vi "Execute Test.vi"(8 "error in (no error)":errorcluster, 9 "Processing":refnum<queue>, 10 "UI in":refnum<queue>, 11 "Settings in":T1 {"Processing Settings"."Test Parameters"."Allowed Tolerance (%) FS" format="%#_4g"; "Acq Settings"."Config Settings"."Simulated Sensor Injection" scale=0.0..100.0}) -> (0 "error out":errorcluster, 2 "UI out":refnum<queue>, 3 "Settings out":T1 {"Processing Settings"."Test Parameters"."Allowed Tolerance (%) FS" format="%#_4g"; "Acq Settings"."Config Settings"."Simulated Sensor Injection" scale=0.0..100.0})   [LabVIEW 2026]
uses:
  controls/UI/Settings Cluster.ctl
  controls/UI/Acq Settings.ctl
  Acquisition/Instrument Specifications Configuration.ctl
  Acquisition/Instrument Specifications Cluster Configuration.ctl
  controls/UI/Measurement Role.ctl
  controls/UI/Config Settings.ctl
  Processing/Processing Settings.ctl
  controls/Messaging Payloads/Sensor CoreData.ctl
  controls/Messaging Payloads/Sensor CoreData Cluster.ctl
  controls/UI/Units Enum.ctl
  controls/UI/Signal Enum.ctl
  Processing/Test Parameters.ctl
  Processing/Test Parameters Cluster.ctl
  controls/UI/Test Sequence Context.ctl
  controls/UI/Direction.ctl
  controls/UI/Session Identfiers.ctl
  controls/UI/Test Sequence Settings.ctl
  controls/UI/Test Sequence State.ctl
  controls/UI/Test Sequence Enum.ctl
  controls/Controller/Stimulus Settings.ctl
  controls/Controller/Stimulus Outputs.ctl
  controls/Controller/Stimulus Output.ctl
  controls/Controller/Controller Core Data.ctl
  controls/Controller/Stimulus Output Configuration.ctl
  controls/Controller/Stimulus Role.ctl
  Architecture/Message Queue/Message Cluster.ctl
  Architecture/Message Queue/Enqueue Message (Single).vi
  Architecture/Message Queue/Message Queue.lvlib
  Settings/Settings.lvlib
  Acquisition/Acquisition.lvlib
  Processing/Processing_Engine.lvlib
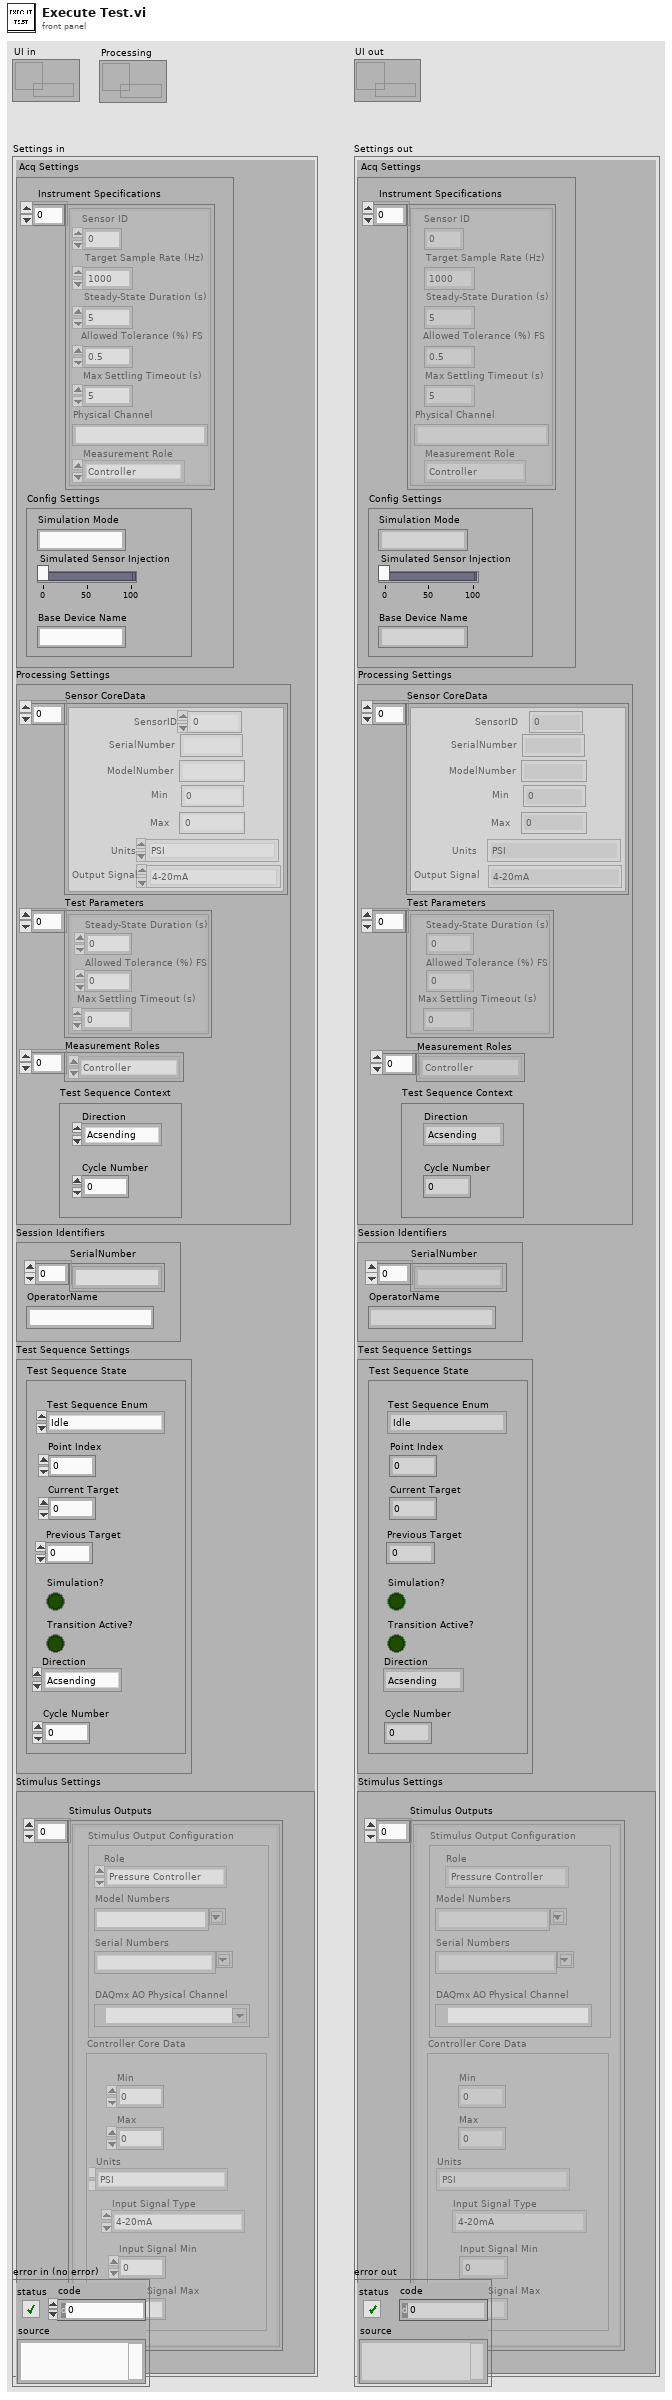
[diagram p1: front panel]
types:
  T1 = typedef "Settings Cluster.ctl" = cluster{"Acq Settings":T2, "Processing Settings":T7, "Session Identifiers":T16, "Test Sequence Settings":T17, "Stimulus Settings":T20}
  T2 = typedef "Acq Settings.ctl" = cluster{"Instrument Specifications":T3, "Config Settings":T6}
  T3 = typedef "Acquisition.lvlib/Instrument Specifications Configuration.ctl" = T4[]
  T4 = typedef "Acquisition.lvlib/Instrument Specifications Cluster Configuration.ctl" = cluster{"Sensor ID":i32, "Target Sample Rate (Hz)":dbl, "Steady-State Duration (s)":i32, "Allowed Tolerance (%) FS":dbl, "Max Settling Timeout (s)":i32, "Physical Channel":string, "Measurement Role":T5}
  T5 = typedef "Settings.lvlib/Measurement Role.ctl" = enum16{"Controller", "Reference", "UUT", "Disable", "All"}
  T6 = typedef "Config Settings.ctl" = cluster{"Simulated Sensor Injection":dbl, "Base Device Name":string, "Simulation Mode":string}
  T7 = typedef "Processing_Engine.lvlib/Processing Settings.ctl" = cluster{"Sensor CoreData":T8, "Test Parameters":T12, "Measurement Roles":T5[], "Test Sequence Context":T14}
  T8 = typedef "Sensor CoreData.ctl" = T9[]
  T9 = typedef "Settings.lvlib/Sensor CoreData Cluster.ctl" = cluster{"SerialNumber":string, "ModelNumber":string, "Min":dbl, "Max":dbl, "Units":T10, "Output Signal":T11, "SensorID":i32}
  T10 = typedef "Units Enum.ctl" = enum16{"PSI", "Deg C", "kPa", "GPM"}
  T11 = typedef "Signal Enum.ctl" = enum16{"4-20mA", "0-10V", "Thermocouple Type K"}
  T12 = typedef "Processing_Engine.lvlib/Test Parameters.ctl" = T13[]
  T13 = typedef "Settings.lvlib/Test Parameters Cluster.ctl" = cluster{"Steady-State Duration (s)":i32, "Allowed Tolerance (%) FS":dbl, "Max Settling Timeout (s)":i32}
  T14 = typedef "Settings.lvlib/Test Sequence Context.ctl" = cluster{"Direction":T15, "Cycle Number":i32}
  T15 = typedef "Settings.lvlib/Direction.ctl" = enum16{"Acsending", "Descending"}
  T16 = typedef "Session Identfiers.ctl" = cluster{"SerialNumber":string[], "OperatorName":string}
  T17 = typedef "Test Sequence Settings.ctl" = cluster{"Test Sequence State":T18}
  T18 = typedef "Settings.lvlib/Test Sequence State.ctl" = cluster{"Test Sequence Enum":T19, "Point Index":i32, "Current Target":dbl, "Previous Target":dbl, "Simulation?":bool, "Direction":T15, "Transition Active?":bool, "Cycle Number":i32}
  T19 = typedef "Test Sequence Enum.ctl" = enum16{"Idle", "Start Point", "Point Complete", "Test Complete", "Abort Test", "Reset"}
  T20 = typedef "Settings.lvlib/Stimulus Settings.ctl" = cluster{"Stimulus Outputs":T21}
  T21 = typedef "Settings.lvlib/Stimulus Outputs.ctl" = T22[]
  T22 = typedef "Settings.lvlib/Stimulus Output.ctl" = cluster{"Controller Core Data":T23, "Stimulus Output Configuration":T24}
  T23 = typedef "Settings.lvlib/Controller Core Data.ctl" = cluster{"Min":dbl, "Max":dbl, "Units":T10, "Input Signal Type":T11, "Input Signal Min":dbl, "Input Signal Max":dbl}
  T24 = typedef "Settings.lvlib/Stimulus Output Configuration.ctl" = cluster{"DAQmx AO Physical Channel":tag, "Role":T25, "Model Numbers":string, "Serial Numbers":string}
  T25 = typedef "Stimulus Role.ctl" = enum16{"Pressure Controller", "Temperature Controller"}
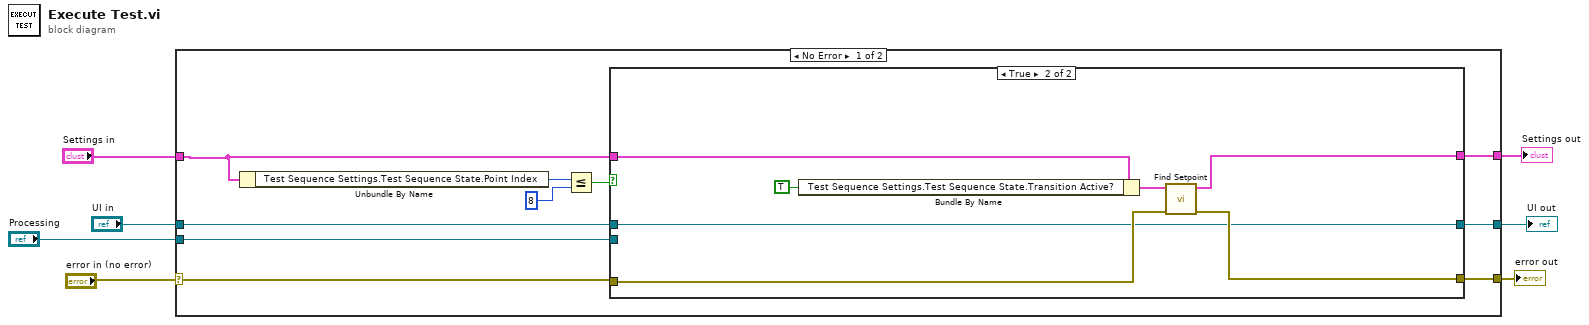
[diagram p0: block diagram]
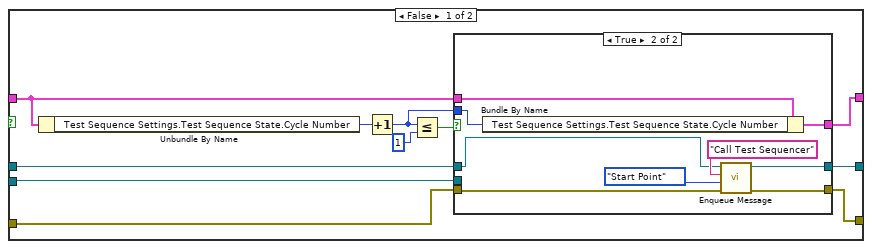
[diagram p2: hidden frame]
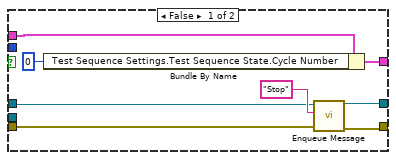
[diagram p3: hidden frame]
diagram:
  n1 = case shown="No Error" "error in (no error)" {
    selector: "error in (no error)" -> [w12 w54]
    tunnel: "Settings in" -> [w9 w55]
    tunnel: [w17 w55] -> w6
    tunnel: [w16 w54] -> w5
    tunnel: "UI in" -> [w11 w53]
    tunnel: [w10 w53] -> w2
    tunnel: "Processing" -> [w8 _]
    frame No Error {
      n2 = Unbundle By Name(w9) -> ("Test Sequence Settings.Test Sequence State.Point Index"=w15:i32)
      n3 = Less Or Equal?(x=w15, y=8) -> (x <= y?=w13:bool)
      n4 = case shown="True" w13 {
        tunnel: w9 -> [w24 w52]
        tunnel: [w22 w49] -> w17
        tunnel: [w26 w48] -> w16
        tunnel: w12 -> [w27 w47]
        tunnel: w11 -> [w28 w46]
        tunnel: [w25 w46] -> w10
        tunnel: w8 -> [w18 _]
        frame False {
          n5 = Unbundle By Name(w24) -> ("Test Sequence Settings.Test Sequence State.Cycle Number"=w23:i32)
          n6 = Increment(x=w23) -> (x+1=w19:i32)
          n7 = Less Or Equal?(x=w19, y=1) -> (x <= y?=w20:bool)
          n8 = case shown="True" w20 {
            tunnel: w28 -> [w35 w38]
            tunnel: w27 -> [w33 w37]
            tunnel: [w32 w44] -> w26
            tunnel: [w34 w43] -> w25
            tunnel: w24 -> [w31 w41]
            tunnel: [w30 w40] -> w22
            tunnel: w19 -> [_ w39]
            tunnel: w18 -> [_ _]
            frame False {
              n9 = Bundle By Name(cluster=w31, "Test Sequence Settings.Test Sequence State.Cycle Number"=0) -> (w30:T1)
              n10 = call-poly "Enqueue Message.vi"("error in (no error)"=w33, "Message"="Stop", "Message Queue"=w35) -> ("error out"=w32:errorcluster, "dup Message Queue"=w34:refnum<queue>)  [unwired: 7 in]
            }
            frame True {
              n11 = Bundle By Name(cluster=w41, "Test Sequence Settings.Test Sequence State.Cycle Number"=w39) -> (w40:T1)
              n12 = call-poly "Enqueue Message.vi"("error in (no error)"=w37, "Message Data"=Test_Sequence_Enum."Start Point" ("Test Sequence Enum"), "Message"="Call Test Sequencer", "Message Queue"=w38) -> ("error out"=w44:errorcluster, "dup Message Queue"=w43:refnum<queue>)  [unwired: 6 in]
            }
          }
        }
        frame True {
          n13 = Bundle By Name(cluster=w52, "Test Sequence Settings.Test Sequence State.Transition Active?"=TRUE) -> (w51:T1)
          n14 = call "Find Setpoint.vi"("error in (no error)"=w47, "Settings in"=w51) -> ("error out"=w48:errorcluster, "Settings out"=w49:T1)  [unwired: 8 in]
        }
      }
    }
    frame Error {
    }
  }
  "Settings out" <- w6
  "error out" <- w5
  "UI out" <- w2
